vi "Do Bar Sample Hall Calculations.vi"(8 "error in (no error)":errorcluster) -> (0 "error out":errorcluster)   [LabVIEW 2016, in "Hall Effect Library.lvlib"]
uses:
  Hall Effect Library.lvlib
  Global Variables/Hall Effect Data.vi
  Global Variables/Test Settings.vi
panel:
  out "uH":dbl
  out "n/p":dbl
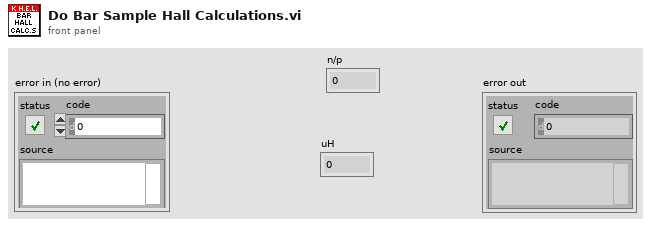
[diagram p1: front panel]
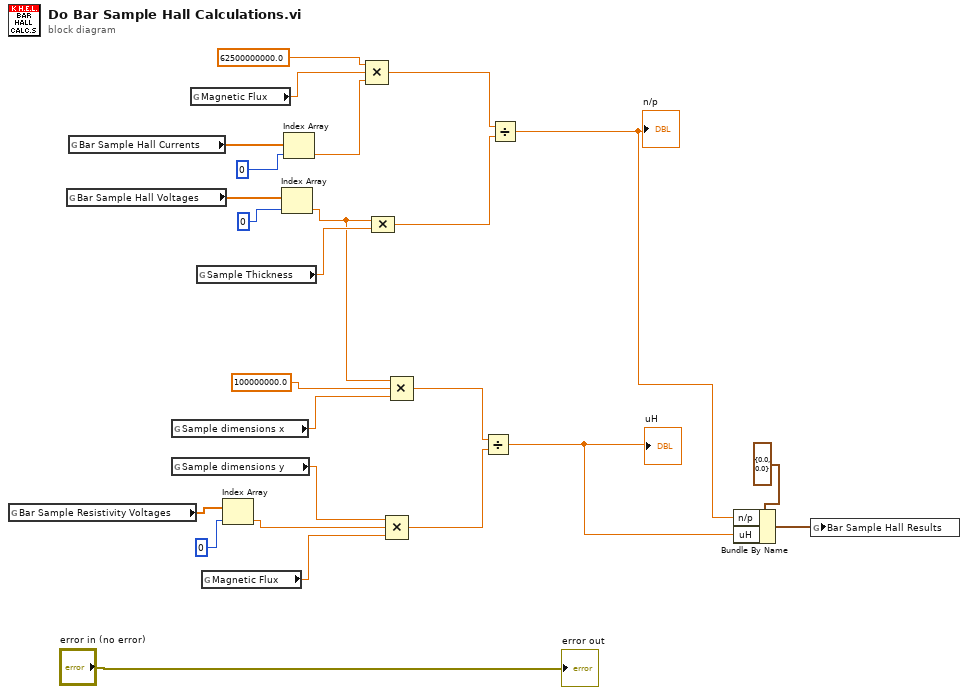
[diagram p0: block diagram]
diagram:
  n1 = global read "Hall Effect Data.vi" "Bar Sample Resistivity Voltages"() -> (w14:dbl[])
  n2 = global read "Hall Effect Data.vi" "Bar Sample Hall Voltages"() -> (w22:dbl[])
  n3 = global read "Hall Effect Data.vi" "Bar Sample Hall Currents"() -> (w24:dbl[])
  n4 = global read "Test Settings.vi" "Sample dimensions x"() -> (w10:dbl)
  n5 = global read "Test Settings.vi" "Sample dimensions y"() -> (w9:dbl)
  n6 = global read "Test Settings.vi" "Magnetic Flux"() -> (w19:dbl)
  n7 = global read "Test Settings.vi" "Sample Thickness"() -> (w17:dbl)
  n8 = global read "Test Settings.vi" "Magnetic Flux"() -> (w7:dbl)
  n9 = Index Array(array=w14, index=0) -> (element=w8:dbl)
  n10 = Index Array(array=w22, index=0) -> (element=w12:dbl)
  n11 = Index Array(array=w24, index=0) -> (element=w18:dbl)
  n12 = Compound Arithmetic op=MULTIPLY(62500000000.0, w19, w18) -> (w16:dbl)
  n13 = Compound Arithmetic op=MULTIPLY(w12, w17) -> (w15:dbl)
  n14 = Compound Arithmetic op=MULTIPLY(w9, w8, w7) -> (w5:dbl)
  n15 = Compound Arithmetic op=MULTIPLY(w12, 100000000.0, w10) -> (w6:dbl)
  n16 = Divide(x=w6, y=w5) -> (x/y=w2:dbl)
  "uH" <- w2
  n17 = Divide(x=w16, y=w15) -> (x/y=w3:dbl)
  "n/p" <- w3
  n18 = Bundle By Name(cluster=cluster{"n/p":dbl, "uH":dbl} {"n/p"=0.0, "uH"=0.0} ("Bar Sample Hall Results"), "n/p"=w3, "uH"=w2) -> (w1:cluster{"n/p":dbl, "uH":dbl})
  n19 = global write "Hall Effect Data.vi" "Bar Sample Hall Results"(w1) -> ()
  "error out" <- "error in (no error)"
